vi "Estudo_aula2.vi"() -> ()   [LabVIEW 2020]
panel:
  in  "Numeric":dbl=15.0
  in  "Knob":dbl(knob) scale=0.0..25.0
  out "Termometro":dbl(slide) caption="Temperatura ambiente" scale=0.0..100.0
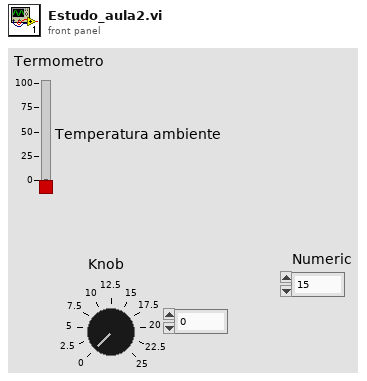
[diagram p1: front panel]
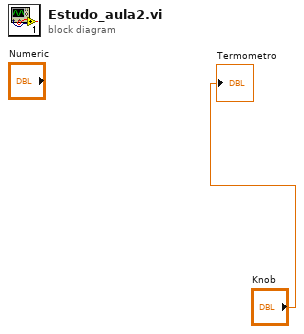
[diagram p0: block diagram]
diagram:
  "Termometro" <- "Knob"
